vi "VI Server_TREE_ClearItemNames.vi"(7 "Label":string, 8 "error in":errorcluster, 9 "Tree.Ref":refnum<vi>, 10 "SingleInstance":bool=TRUE, 11 "VI Server.RefsCluster":T1) -> (0 "error out":errorcluster, 1 "Tree.Ref.DUP":refnum<vi>, 3 "VI Server.RefsCluster.DUP":T1)   [LabVIEW 2020]
uses:
  VI Server_TypeDefs/VI Server_RefsCluster.ctl
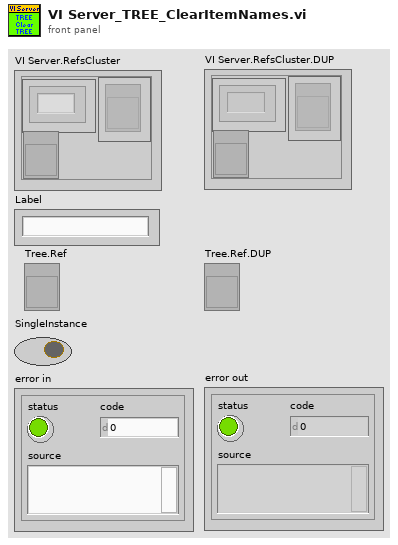
[diagram p1: front panel]
types:
  T1 = typedef "VI Server_RefsCluster.ctl" = cluster{"Labels":string[], "Refs":refnum<vi>[], "VI Ref":refnum<vi>}
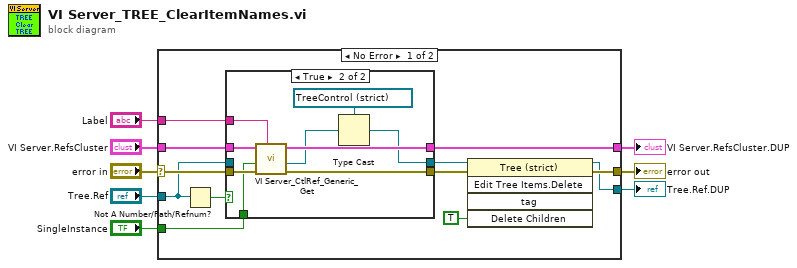
[diagram p0: block diagram]
diagram:
  n1 = case shown="No Error" "error in" {
    selector: "error in" -> [w20 w34]
    tunnel: [w12 w34] -> w7
    tunnel: "VI Server.RefsCluster" -> [w19 w33]
    tunnel: [w18 w33] -> w5
    tunnel: "Label" -> [w17 _]
    tunnel: "SingleInstance" -> [w16 _]
    tunnel: [w11 _] -> w2
    tunnel: "Tree.Ref" -> [w9 _]
    frame No Error {
      n2 = Not A Number/Path/Refnum?(number/path/refnum=w9) -> (NaN/Path/Refnum?=w10:bool)
      n3 = case shown="True" w10 {
        tunnel: w20 -> [w23 w32]
        tunnel: w19 -> [w21 w31]
        tunnel: [w21 w30] -> w18
        tunnel: w17 -> [_ w29]
        tunnel: w16 -> [_ w27]
        tunnel: [w22 w25] -> w14
        tunnel: [w23 w24] -> w13
        tunnel: w9 -> [w22 _]
        frame False {
        }
        frame True {
          n4 = call "VI Server_CtlRef_Generic_Get.vi"("Control.Label"=w29, "error in"=w32, "SingleInstance"=w27, "VI Server.RefsCluster"=w31) -> ("error out"=w24:errorcluster, "Control.Ref.Generic"=w28:refnum<vi>, "VI Server.RefsCluster.DUP"=w30:T1)  [unwired: 5 in]
          n5 = Type Cast(type=refnum<vi> refnum ("Tree"), x=w28) -> (*(type *) &x=w25:refnum<vi>)
        }
      }
      n6 = invoke on="Invoke Node" class="Tree (strict)" method="Edit Tree Items.Delete"(reference=w14, error in=w13, "Delete Children"=TRUE ("Delete Children?")) -> (reference out=w11:refnum<vi>, error out=w12:errorcluster)  [unwired: 2 in, 3 out]
    }
    frame Error {
    }
  }
  "VI Server.RefsCluster.DUP" <- w5
  "error out" <- w7
  "Tree.Ref.DUP" <- w2
